vi "Read Totalizer.vi"(0 "VISA resource name":refnum<visa-resource-name>="GPIB0::16::INSTR", 5 "Totalizer Channel (125)":string="125", 11 "error in (no error)":errorcluster) -> (4 "VISA resource name out":refnum<visa-resource-name>, 6 "Totalizer Count":i32, 15 "error out":errorcluster)   [LabVIEW 2020, in "Keithley 27XX.lvlib"]
doc: "This VI returns the current Totalizer Count on a slected Totalizer Channel. Use Configure Totalizer.vi to configure events triggered by this VI.\n\nNote\n(1) The Model 77xx card being used must have Totalizer support. \n\n(2) On the 7706 Multiplexer Card there is one totalizer channel - Ch 25"
uses:
  Keithley 27XX.lvlib
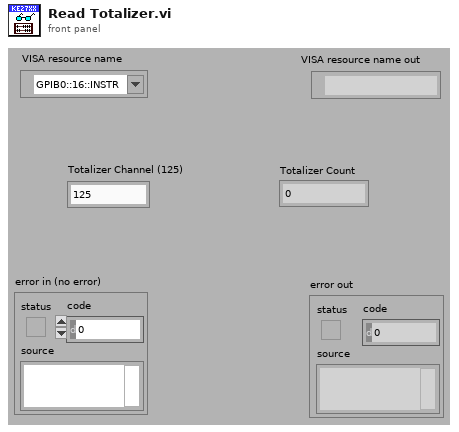
[diagram p1: front panel]
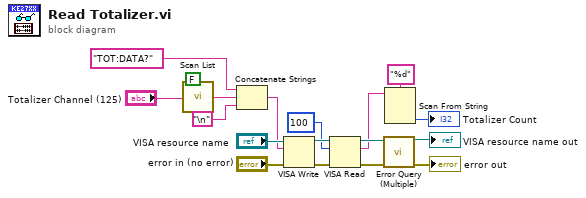
[diagram p0: block diagram]
diagram:
  n1 = call "Scan List.vi"("Add Comma (True)"=FALSE ("Comma? (True)"), "Scan List (Empty)"="Totalizer Channel (125)") -> ("Scan List Out"=w14:string)  [unwired: 13 in]
  n2 = Concatenate Strings("TOT:DATA?", w14, "\n") -> (w12:string)
  n3 = VISA Write(VISA resource name="VISA resource name", write buffer=w12, error in (no error)="error in (no error)") -> (VISA resource name out=w11:refnum<visa-resource-name>, error out=w10:errorcluster)  [unwired: 1 out]
  n4 = VISA Read(VISA resource name=w11, byte count=u32 100, error in (no error)=w10) -> (VISA resource name out=w5:refnum<visa-resource-name>, read buffer=w3:string, error out=w6:errorcluster)  [unwired: 1 out]
  n5 = call "Error Query (Multiple).vi"("VISA resource name"=w5, "error in (no error)"=w6) -> ("VISA resource name out"=→"VISA resource name out":refnum<visa-resource-name>, "error out"=→"error out":errorcluster)  [unwired: 10 in, 2 out]
  n6 = Scan From String(format string="%d", input string=w3) -> (output 1=→"Totalizer Count":i32)  [unwired: 3 in, 3 out]
